vi "Get Report Type.vi"(0 "report in":refnum<class "NI_report.lvclass">, 11 "error in (no error)":errorcluster) -> (4 "report out":refnum<class "NI_report.lvclass">, 8 "report type":T1(ring)=enum."HTML", 15 "error out":errorcluster)   [LabVIEW 2017, in "NI_report.lvclass"]
doc: "Returns the report type, such as standard on Windows, or HTML on all platforms, of a specified report.\n\nThis VI also returns Microsoft Word or Excel report types."
uses:
  <vilib>/Utility/NIReport.llb/NI_report.lvclass
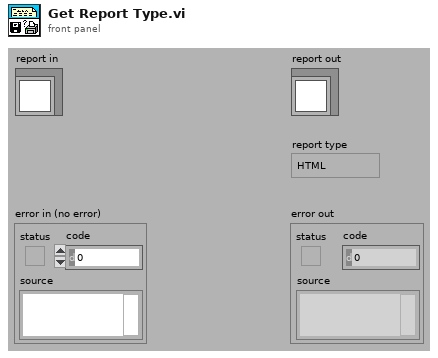
[diagram p1: front panel]
types:
  T1 = enum16{"Standard Report", "HTML", "Word", "Excel"}
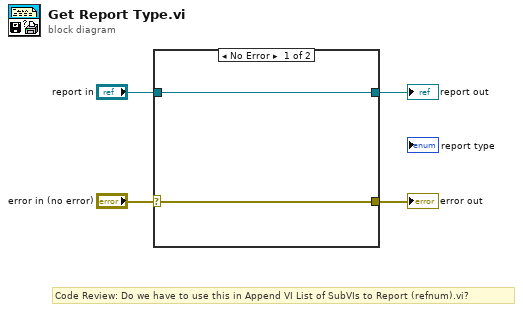
[diagram p0: block diagram]
diagram:
  # "Code Review: Do we have to use this in Append VI List of SubVIs to Report (refnum).vi?"
  n1 = case shown="No Error" "error in (no error)" {
    selector: "error in (no error)" -> [w6 w8]
    tunnel: [w6 w8] -> w3
    tunnel: [w5 w7] -> w1
    tunnel: "report in" -> [w5 w7]
    frame No Error {
    }
    frame Error {
    }
  }
  "error out" <- w3
  "report out" <- w1
